vi "Hamburger Basic Example.vi"() -> ()   [LabVIEW 2017]
uses:
  HamburgerMenu/HamburgerMenu.lvclass
panel:
  out "Title":string="Hamburger Button Test VI"
  in  "Menu Button":bool
  out "HamburgerItemClicked":string
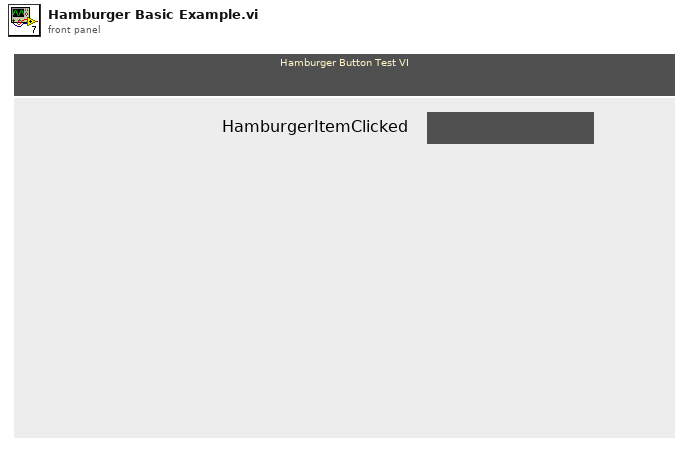
[diagram p1: front panel]
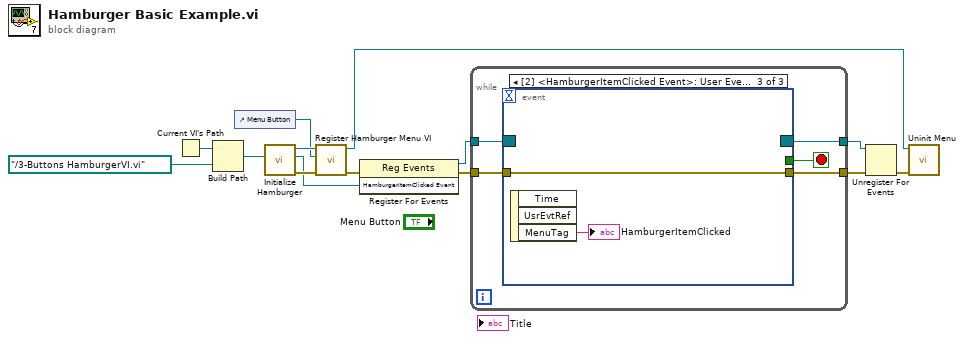
[diagram p0: block diagram]
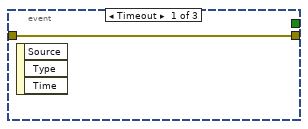
[diagram p2: hidden frame]
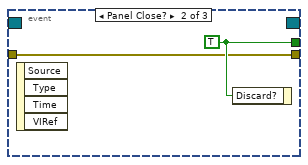
[diagram p3: hidden frame]
diagram:
  n1 = Current VI's Path() -> (path=w14:path)
  n2 = Build Path(base path=w14, name or relative path=path "../3-Buttons HamburgerVI.vi") -> (appended path=w8:path)
  n3 = control-ref of="Menu Button"() -> (w4:refnum<vi>)
  n4 = call "Initialize Hamburger.vi"("MenuVI Path"=w8) -> ("error out"=w10:errorcluster, "HamburgerItemClicked Event"=w7:refnum<user-event>, "HamburgerMenu Obj"=w9:refnum<class "HamburgerMenu.lvclass">)  [unwired: 8 in]
  n5 = call "Register Hamburger Menu VI.vi"("error in (no error)"=w10, "Hamburger Support Control Refnum"=w4, "HamburgerMenu Obj in"=w9) -> ("error out"=w3:errorcluster, "HamburgerMenu Obj"=w13:refnum<class "HamburgerMenu.lvclass">)  [unwired: 7 in]
  n6 = register-events(error in=w3, w7) -> (reference out=w6:refnum<event-registration>, error out=w1:errorcluster)  [unwired: 1 in]
  n7 = while {
    tunnel: [w18] -> w12
    tunnel: w6 -> [w17]
    tunnel: [w16] -> w2
    tunnel: w1 -> [w15]
    stop <- w19 stop-if-true
    n8 = event shown="[2] <HamburgerItemClicked Event>: User Event" {
      selector: w17 -> [_ _ _]
      dyn-events: [_ _ _] -> w18
      timeout: _ -> [_ _ _]
      tunnel: [_ w22 _] -> w19
      tunnel: [w20 w21 w23] -> w16
      tunnel: w15 -> [w20 w21 w23]
      event Timeout {
        n9 = event-data() -> ()  [unwired: 1 in, 3 out]
      }
      event Panel Close? {
        w22 = TRUE ("Discard?")
        n10 = event-data() -> ()  [unwired: 1 in, 4 out]
        n11 = event-data("Discard?"=w22) -> ()  [unwired: 1 in, 1 out]
      }
      event User Event {
        n12 = event-data() -> ("MenuTag"=→"HamburgerItemClicked":string)  [unwired: 1 in, 2 out]
      }
    }
  }
  n13 = Unregister For Events(event registration refnum=w12, error in=w2) -> (error out=w11:errorcluster)
  n14 = call "Uninit Menu.vi"("error in (no error)"=w11, "HamburgerMenu in"=w13) -> ()  [unwired: 8 in, 2 out]
